vi "Parse Tree Management Data.vi"(3 "Tree Menu Data":T2[](array[typedef])) -> (1 "Array":T1(array[cluster]))   [LabVIEW 2020, in "Config Data.lvlib" / "Config Data.lvclass"]
uses:
  Config Data.lvclass
  Config Data.lvclass/Config Data.ctl
  typedefs/Tree Menu Entry.ctl
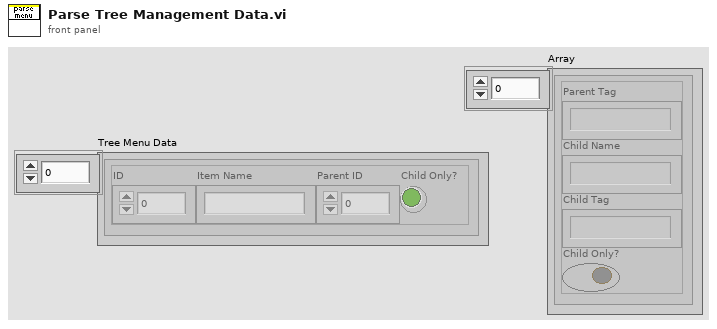
[diagram p1: front panel]
types:
  T1 = cluster{"Parent Tag":string, "Child Name":string, "Child Tag":string, "Child Only?":bool}[]
  T2 = typedef "Config Data.lvlib/Config Data.lvclass/Tree Menu Entry.ctl" = cluster{"ID":i32, "Item Name":string, "Parent ID":i32, "Child Only?":bool}
  T3 = cluster{"Parent Tag":string, "Child Name":string, "Child Tag":string, "Child Only?":bool}
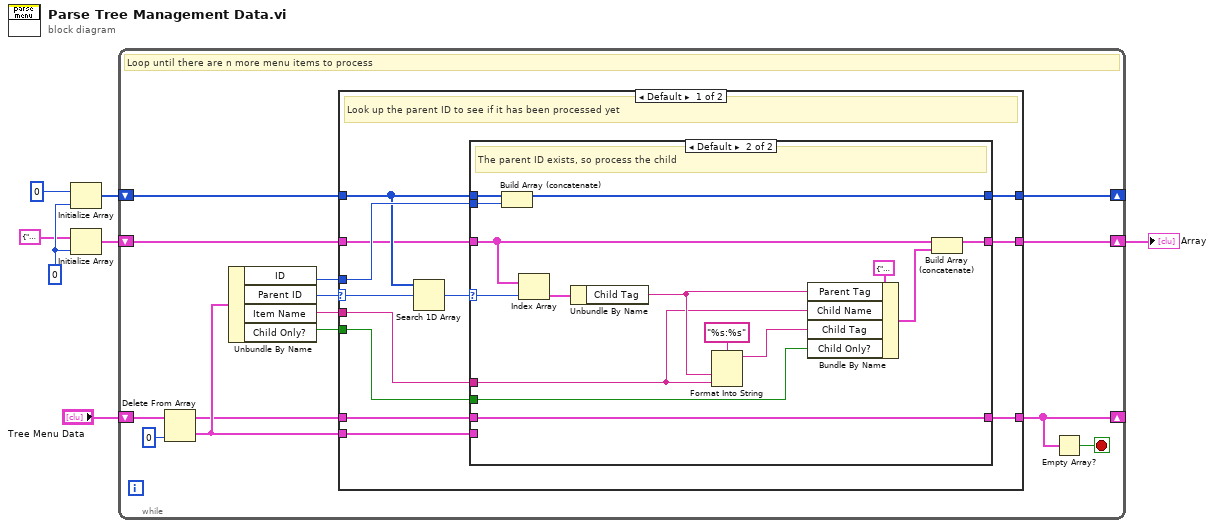
[diagram p0: block diagram]
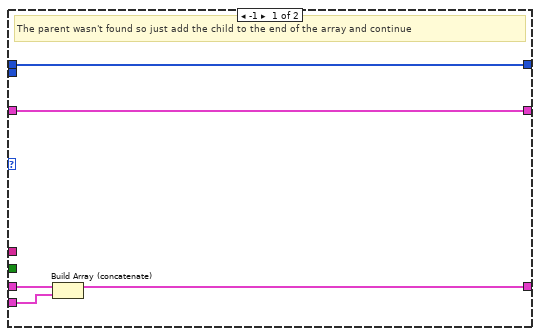
[diagram p2: hidden frame]
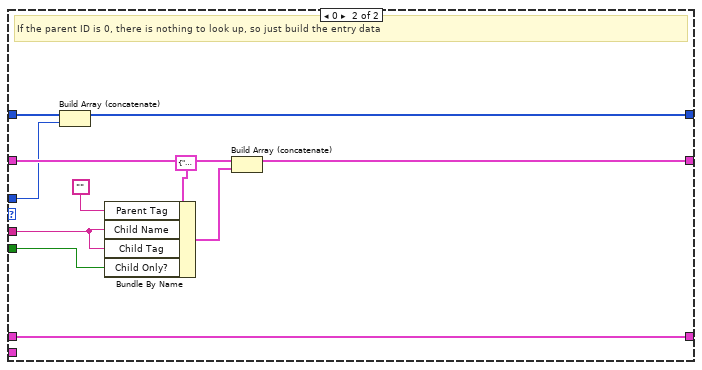
[diagram p3: hidden frame]
diagram:
  w4 = 0 ("dimension size")
  n1 = Initialize Array(0 ("dimension size"), w4) -> (w3:i32[])
  n2 = Initialize Array(T3 {"Parent Tag"="", "Child Name"="", "Child Tag"="", "Child Only?"=FALSE}, w4) -> (w1:T1)
  n3 = while {
    shift-right: [w18] -> w6
    shift-left: w1 -> [w19]
    shift-right: [w16] -> _
    shift-left: w3 -> [w17]
    shift-right: [w10] -> _
    shift-left: "Tree Menu Data" -> [w14]
    stop <- w9 stop-if-true
    # "Loop until there are n more menu items to process"
    n4 = Delete From Array(array=w14, index=0) -> (deleted portion=w12:T2, array with subset deleted=w11:T2[])  [unwired: 1 in]
    n5 = Unbundle By Name(w12) -> ("ID"=w20:i32, "Parent ID"=w15:i32, "Item Name"=w21:string, "Child Only?"=w8:bool)
    n6 = case shown="Default" w15 {
      selector: w15 -> [w30 _]
      tunnel: w21 -> [w26 w61]
      tunnel: w20 -> [w31 w56]
      tunnel: w19 -> [w27 w64]
      tunnel: [w33 w63] -> w18
      tunnel: w17 -> [w29 w58]
      tunnel: [w32 w57] -> w16
      tunnel: w12 -> [w24 _]
      tunnel: w11 -> [w25 w55]
      tunnel: [w23 w55] -> w10
      tunnel: w8 -> [w22 w54]
      frame Default {
        # "Look up the parent ID to see if it has been processed yet"
        n7 = Search 1D Array(1D array=w29, element=w30) -> (index of element=w28:i32)  [unwired: 1 in]
        n8 = case shown="Default" w28 {
          selector: w28 -> [_ w47]
          tunnel: [w37 w53] -> w33
          tunnel: [w38 w52] -> w32
          tunnel: w31 -> [_ w51]
          tunnel: w29 -> [w38 w48]
          tunnel: w27 -> [w37 w46]
          tunnel: w26 -> [_ w42]
          tunnel: w25 -> [w36 w40]
          tunnel: w24 -> [w35 _]
          tunnel: [w34 w40] -> w23
          tunnel: w22 -> [_ w39]
          frame -1 {
            # "The parent wasn't found so just add the child to the end of the array and continue"
            n9 = Build Array (concatenate)(w36, w35) -> (w34:T2[])
          }
          frame Default {
            # "The parent ID exists, so process the child"
            n10 = Build Array (concatenate)(w48, w51) -> (w52:i32[])
            n11 = Index Array(array=w46, index=w47) -> (element=w45:T3)
            n12 = Unbundle By Name(w45) -> ("Child Tag"=w43:string)
            n13 = Format Into String(format string="%s:%s", w43, w42) -> (resulting string=w44:string)  [unwired: 2 in, 1 out]
            n14 = Bundle By Name(cluster=T3 {"Parent Tag"="", "Child Name"="", "Child Tag"="", "Child Only?"=FALSE}, "Parent Tag"=w43, "Child Name"=w42, "Child Tag"=w44, "Child Only?"=w39) -> (w49:T3)
            n15 = Build Array (concatenate)(w46, w49) -> (w53:T1)
          }
        }
      }
      frame 0 {
        # "If the parent ID is 0, there is nothing to look up, so just build the entry data"
        n16 = Build Array (concatenate)(w58, w56) -> (w57:i32[])
        n17 = Bundle By Name(cluster=T3 {"Parent Tag"="", "Child Name"="", "Child Tag"="", "Child Only?"=FALSE}, "Parent Tag"="", "Child Name"=w61, "Child Tag"=w61, "Child Only?"=w54) -> (w59:T3)
        n18 = Build Array (concatenate)(w64, w59) -> (w63:T1)
      }
    }
    n19 = Empty Array?(array=w10) -> (empty?=w9:bool)
  }
  "Array" <- w6
